vi "Menu Building Initialization Merge VI.vi"   [LabVIEW 2016]
doc: "This Merge VI is a good starting place for most MenuBuilding menus. It has all of the vi's needed to initialize a new menu"
uses:
  <userlib>/_MGI/Menu Building/MenuTypes/MGI_Menu.lvclass
  <userlib>/_MGI/Menu Building/MenuItem/MGI_MenuItem.lvclass
  <userlib>/_MGI/Menu Building/MenuItem/MenuItem.vi
  <userlib>/_MGI/Menu Building/MenuTypes/Vi/VI.vi
  <userlib>/_MGI/Menu Building/MenuTypes/Vi/MGI_VI.lvclass
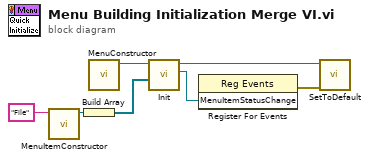
[diagram p0: block diagram]
diagram:
  n1 = call-poly <userlib>:"MenuItemConstructor.vi"("Text"="File") -> ("MenuItem"=w1:refnum<data-value>)  [unwired: 9 in, 1 out]
  n2 = Build Array(w1) -> (w4:refnum<data-value>[])
  n3 = call-poly <userlib>:"MenuConstructor.vi"() -> ("VI"=w3:refnum<class "MGI_VI.lvclass">)  [unwired: 10 in, 1 out]
  n4 = call-dynamic "Init.vi"("Menu Items"=w4, "Menu in"=w3) -> ("MenuItemStatusChange"=w7:refnum<user-event>, "Menu out"=w6:refnum<class "MGI_VI.lvclass">)  [unwired: 7 in, 1 out]
  n5 = register-events(w7) -> (error out=w5:errorcluster)  [unwired: 2 in, 1 out]
  n6 = call-dynamic "SetToDefault.vi"("error in (no error)"=w5, "Menu in"=w6) -> ()  [unwired: 8 in, 2 out]
